vi "Tusk.GetTuskFromDictionary.vi"(8 "error in (no error)":errorcluster, 10 "Name (Local)":string, 11 "Tusk in":refnum<class "Tusk.lvclass">) -> (0 "error out":errorcluster, 2 "Tusk":refnum<class "Tusk.lvclass">, 3 "Tusk out":refnum<class "Tusk.lvclass">)   [LabVIEW 2018, in "Application.lvlib" / "Tusk.lvclass"]
uses:
  Tusk.lvclass
  Tusk.lvclass/Tusk.ctl
  Dictionary Class/Dictionary.lvclass/Dictionary.ctl
  3fa77438-33e4-48e7-a501-c74b9750b9f8.vi
  bb4b4b2f-5120-4767-9776-c61ed956de36.vi
  Dictionary Class/VIs/Get Data DVR.vi
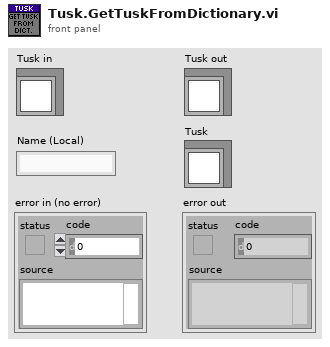
[diagram p1: front panel]
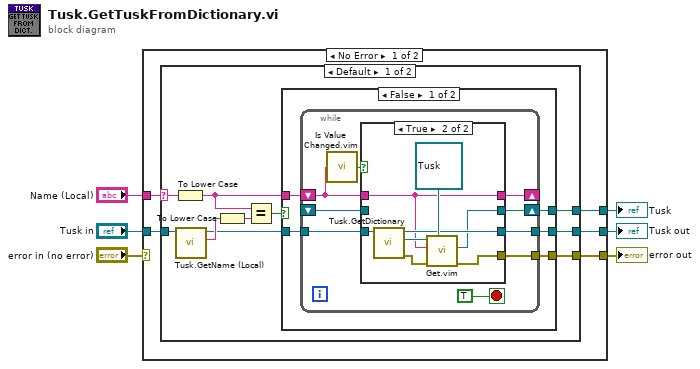
[diagram p0: block diagram]
diagram:
  n1 = case shown="No Error" "error in (no error)" {
    selector: "error in (no error)" -> [_ w50]
    tunnel: [w7 w50] -> w5
    tunnel: [w9 w49] -> w3
    tunnel: "Tusk in" -> [w10 w49]
    tunnel: "Name (Local)" -> [w11 _]
    tunnel: [w8 _] -> w1
    frame No Error {
      n2 = case shown="Default" w11 {
        selector: w11 -> [w20 _]
        tunnel: w10 -> [w21 w48]
        tunnel: [w14 w48] -> w9
        tunnel: [w13 w48] -> w8
        tunnel: [w12 _] -> w7
        frame Default {
          n3 = To Lower Case(string=w20) -> (all lower case string=w15:string)
          n4 = call "Tusk.GetName (Local).vi"("Tusk in"=w21) -> ("Name(Local)"=w19:string, "Tusk out"=w16:refnum<class "Tusk.lvclass">)  [unwired: 8 in, 1 out]
          n5 = To Lower Case(string=w19) -> (all lower case string=w18:string)
          n6 = Equal?(x=w15, y=w18) -> (x = y?=w17:bool)
          n7 = case shown="False" w17 {
            tunnel: w16 -> [w26 w47]
            tunnel: w15 -> [w24 _]
            tunnel: [w25 w47] -> w14
            tunnel: [w23 w47] -> w13
            tunnel: [w22 _] -> w12
            frame False {
              n8 = while {
                shift-right: [w31] -> _
                shift-left: w24 -> [w30]
                shift-right: [w33] -> w23
                shift-left: _ -> [w29]
                tunnel: w26 -> [w35]
                tunnel: [w34] -> w25
                tunnel: [w27] -> w22
                stop <- TRUE stop-if-true
                n9 = call "Is Value Changed.vim"("value"=w30) -> ("changed or first call?"=w32:bool)
                n10 = case shown="False" w32 {
                  tunnel: w35 -> [w38 w43]
                  tunnel: [w38 w42] -> w34
                  tunnel: [w37 w41] -> w33
                  tunnel: w30 -> [w36 w39]
                  tunnel: [w36 w39] -> w31
                  tunnel: w29 -> [w37 _]
                  tunnel: [_ w40] -> w27
                  frame False {
                  }
                  frame True {
                    n11 = call "Tusk.GetDictionary.vi"("Tusk in"=w43) -> ("error out"=w44:errorcluster, "Dictionary"=w46:refnum<class "Dictionary.lvclass">, "Tusk out"=w42:refnum<class "Tusk.lvclass">)  [unwired: 8 in]
                    n12 = call "Get.vim"("Type/Default"=refnum<class "Tusk.lvclass"> refnum ("Tusk out"), "error in (no error)"=w44, "Key"=w39, "Dictionary in"=w46) -> ("error out"=w40:errorcluster, "Value"=w41:refnum<class "Tusk.lvclass">)  [unwired: 4 in, 2 out]
                  }
                }
              }
            }
            frame True {
            }
          }
        }
        frame "{Self}" {
        }
      }
    }
    frame Error {
    }
  }
  "error out" <- w5
  "Tusk out" <- w3
  "Tusk" <- w1
